vi "Acquire Data using 5772 (DRAM_200fifo_110M_globals).vi"() -> ()   [LabVIEW 2012]
uses:
  <vilib>/Platform/TimedLoop/XDataNode/XDataNode.xnode
  <vilib>/Platform/TimedLoop/XDataNode/nitl_modes.ctl
  <vilib>/Platform/TimedLoop/XDataNode/XDNodeRunTimeDep.lvlib
  <vilib>/Platform/TimedLoop/XDataNode/wakeup.ctl
  <vilib>/Platform/TimedLoop/XDataNode/timing_clust.ctl
  <vilib>/rvi/FXPMathLib/basic elements/FxpDiscreteDelay/XNode/nifxpmath_DiscreteDelay.xnode
  <userlib>/FPGA Library/Code Development/DRAM/RF-RIO/FIFO/FIFO/FPGA/FIFO.lvlib
  <userlib>/Fast OCT/Debug/Version 1/Channel Data/Data from Channel 0 and Channel 1.vi
  <userlib>/Fast OCT/Debug/Version 1/Globals/Controls.vi
panel:
  out "Record Count":u32
  out "U256s from DRAM FIFO":u32
  out "U256s to DRAM FIFO":u32
  out "Host FIFO Timed Out?":bool
  out "U64s to Host":u32
  out "U256s Acquired":u32
  in  "DRAM Arbiter Config":T1={"write grant time (clocks)"=256, "read grant time (clocks)"=256}
  in  "DRAM FIFO Depth":u8(ring)=20 items=["4"=2, "8"=3, "16"=4, "32"=5, "64"=6, "128"=7, "256"=8, "512"=9, "1024"=10, "2048"=11, "4096"=12, "8192"=13, "16384"=14, "32768"=15, "65536"=16, "131072"=17, "262144"=18, "524288"=19, "1048576"=20, "2097152"=21, "4194304"=22, "8388608"=23, "16777216"=24, "33554432"=25, "67108864"=26, "134217728"=27, "268435456"=28, "536870912"=29, "1073741824"=30, "2147483648"=31, "4294967296"=32]
  in  "Record Parameters":T2={"Load Record Parameters?"=FALSE, "Pre Trigger Samples"=2, "Post Trigger Samples"=1000, "Trigger Hold Off"=0, "Record Count"=1} {"Pre Trigger Samples" min=2}
  out "IO Module Status":T3
  out "Buffer Timed Out?":bool
  in  "Software Trigger":bool
  in  "Trigger Type":T4(ring)=enum."Software Trigger"
  in  "Arm Acquisition Engine":bool
  # "Digitial Trigger Input:\nPXI_Trig0 or DIO 0 on CB Front Panel"
  # "Interactive Mode Instructions\n1) Run the Emulation Mode VI for Stimulus\n1) Click on acq.Initiate, First to False and Then to True\n2) Click on Host Trigger"
  # "Status"
  # "Acquisition Engine"
  # "Acquisition Status"
  # "Record Parameters"
  # "Memory Configuration"
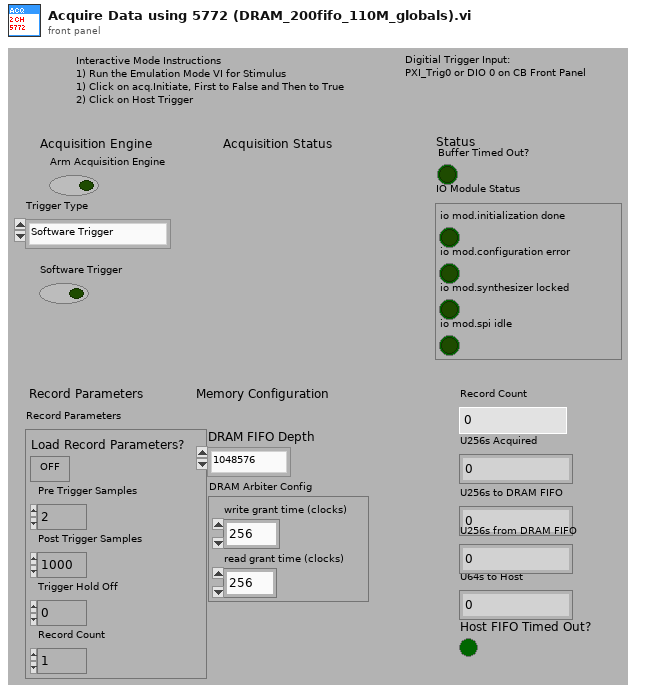
[diagram p1: front panel]
types:
  T1 = cluster{"write grant time (clocks)":u16, "read grant time (clocks)":u16}
  T2 = cluster{"Load Record Parameters?":bool, "Pre Trigger Samples":u32, "Post Trigger Samples":u32, "Trigger Hold Off":u32, "Record Count":u32}
  T3 = cluster{"io mod.initialization done":bool, "io mod.configuration error":bool, "io mod.synthesizer locked":bool, "io mod.spi idle":bool}
  T4 = enum8{"Immediate Trigger", "Software Trigger", "External Digital Trigger", "Analog Trigger"}
  T5 = typedef "XDNodeRunTimeDep.lvlib/timing_clust.ctl" = cluster{"Expected End [f-1]":u64, "Actual End [f-1]":u64, "Finished Late? [f-1]":bool, "Expected End [i-1]":u64, "Actual End [i-1]":u64, "Finished Late? [i-1]":bool, "Expected Start [i]":u64, "Actual Start [i]":u64, "Expected Start [f]":u64, "Actual Start [f]":u64, "Source Name":string, "Structure Name":string, "Period":i64, "Deadline":i64, "Offset":i64, "Start":i64, "Priority":i32, "Timeout":i32, "Mode":T6, "Wakeup Reason":T7, "Error":errorcluster, "Source Type":string, "Secondary Source Type":string, "Global End Time":u64, "Global Start Time":u64, "Frame Duration":u64, "Iteration Duration":u64, "Assigned CPU":i32, "I/O Scan Engine Mode":u32}
  T6 = typedef "XDNodeRunTimeDep.lvlib/nitl_modes.ctl" = enum32{"No Change", "Process missed periods, maintain original phase", "Discard missed periods, maintain original phase", "Process missed periods, ignore original phase", "Discard missed periods, ignore original phase"}
  T7 = typedef "XDNodeRunTimeDep.lvlib/wakeup.ctl" = enum32{"Normal", "Aborted", "Asynchronous wakeup", "Timing source error", "Timed loop error", "Timeout"}
  T8 = cluster{"fifo1 memory":refnum<k21>, "fifo2 memory":refnum<k21>}
  T9 = cluster{"Data 0":u64, "Data 1":u64, "Data 2":u64, "Data 3":u64}
  T10 = cluster{"Output":cluster{"Data 0":u64, "Data 1":u64, "Data 2":u64, "Data 3":u64}, "Output Valid":bool}
  T11 = typedef "Data Type (256).ctl" = cluster{"Bank0. High":u64, "Bank0. Low":u64, "Bank1. High":u64, "Bank1. Low":u64}
  T12 = typedef "acqEngineStates v1.ctl" = cluster{"Triggered":bool, "TrigArmed":bool, "RdyForArm":bool, "Reserved":bool}
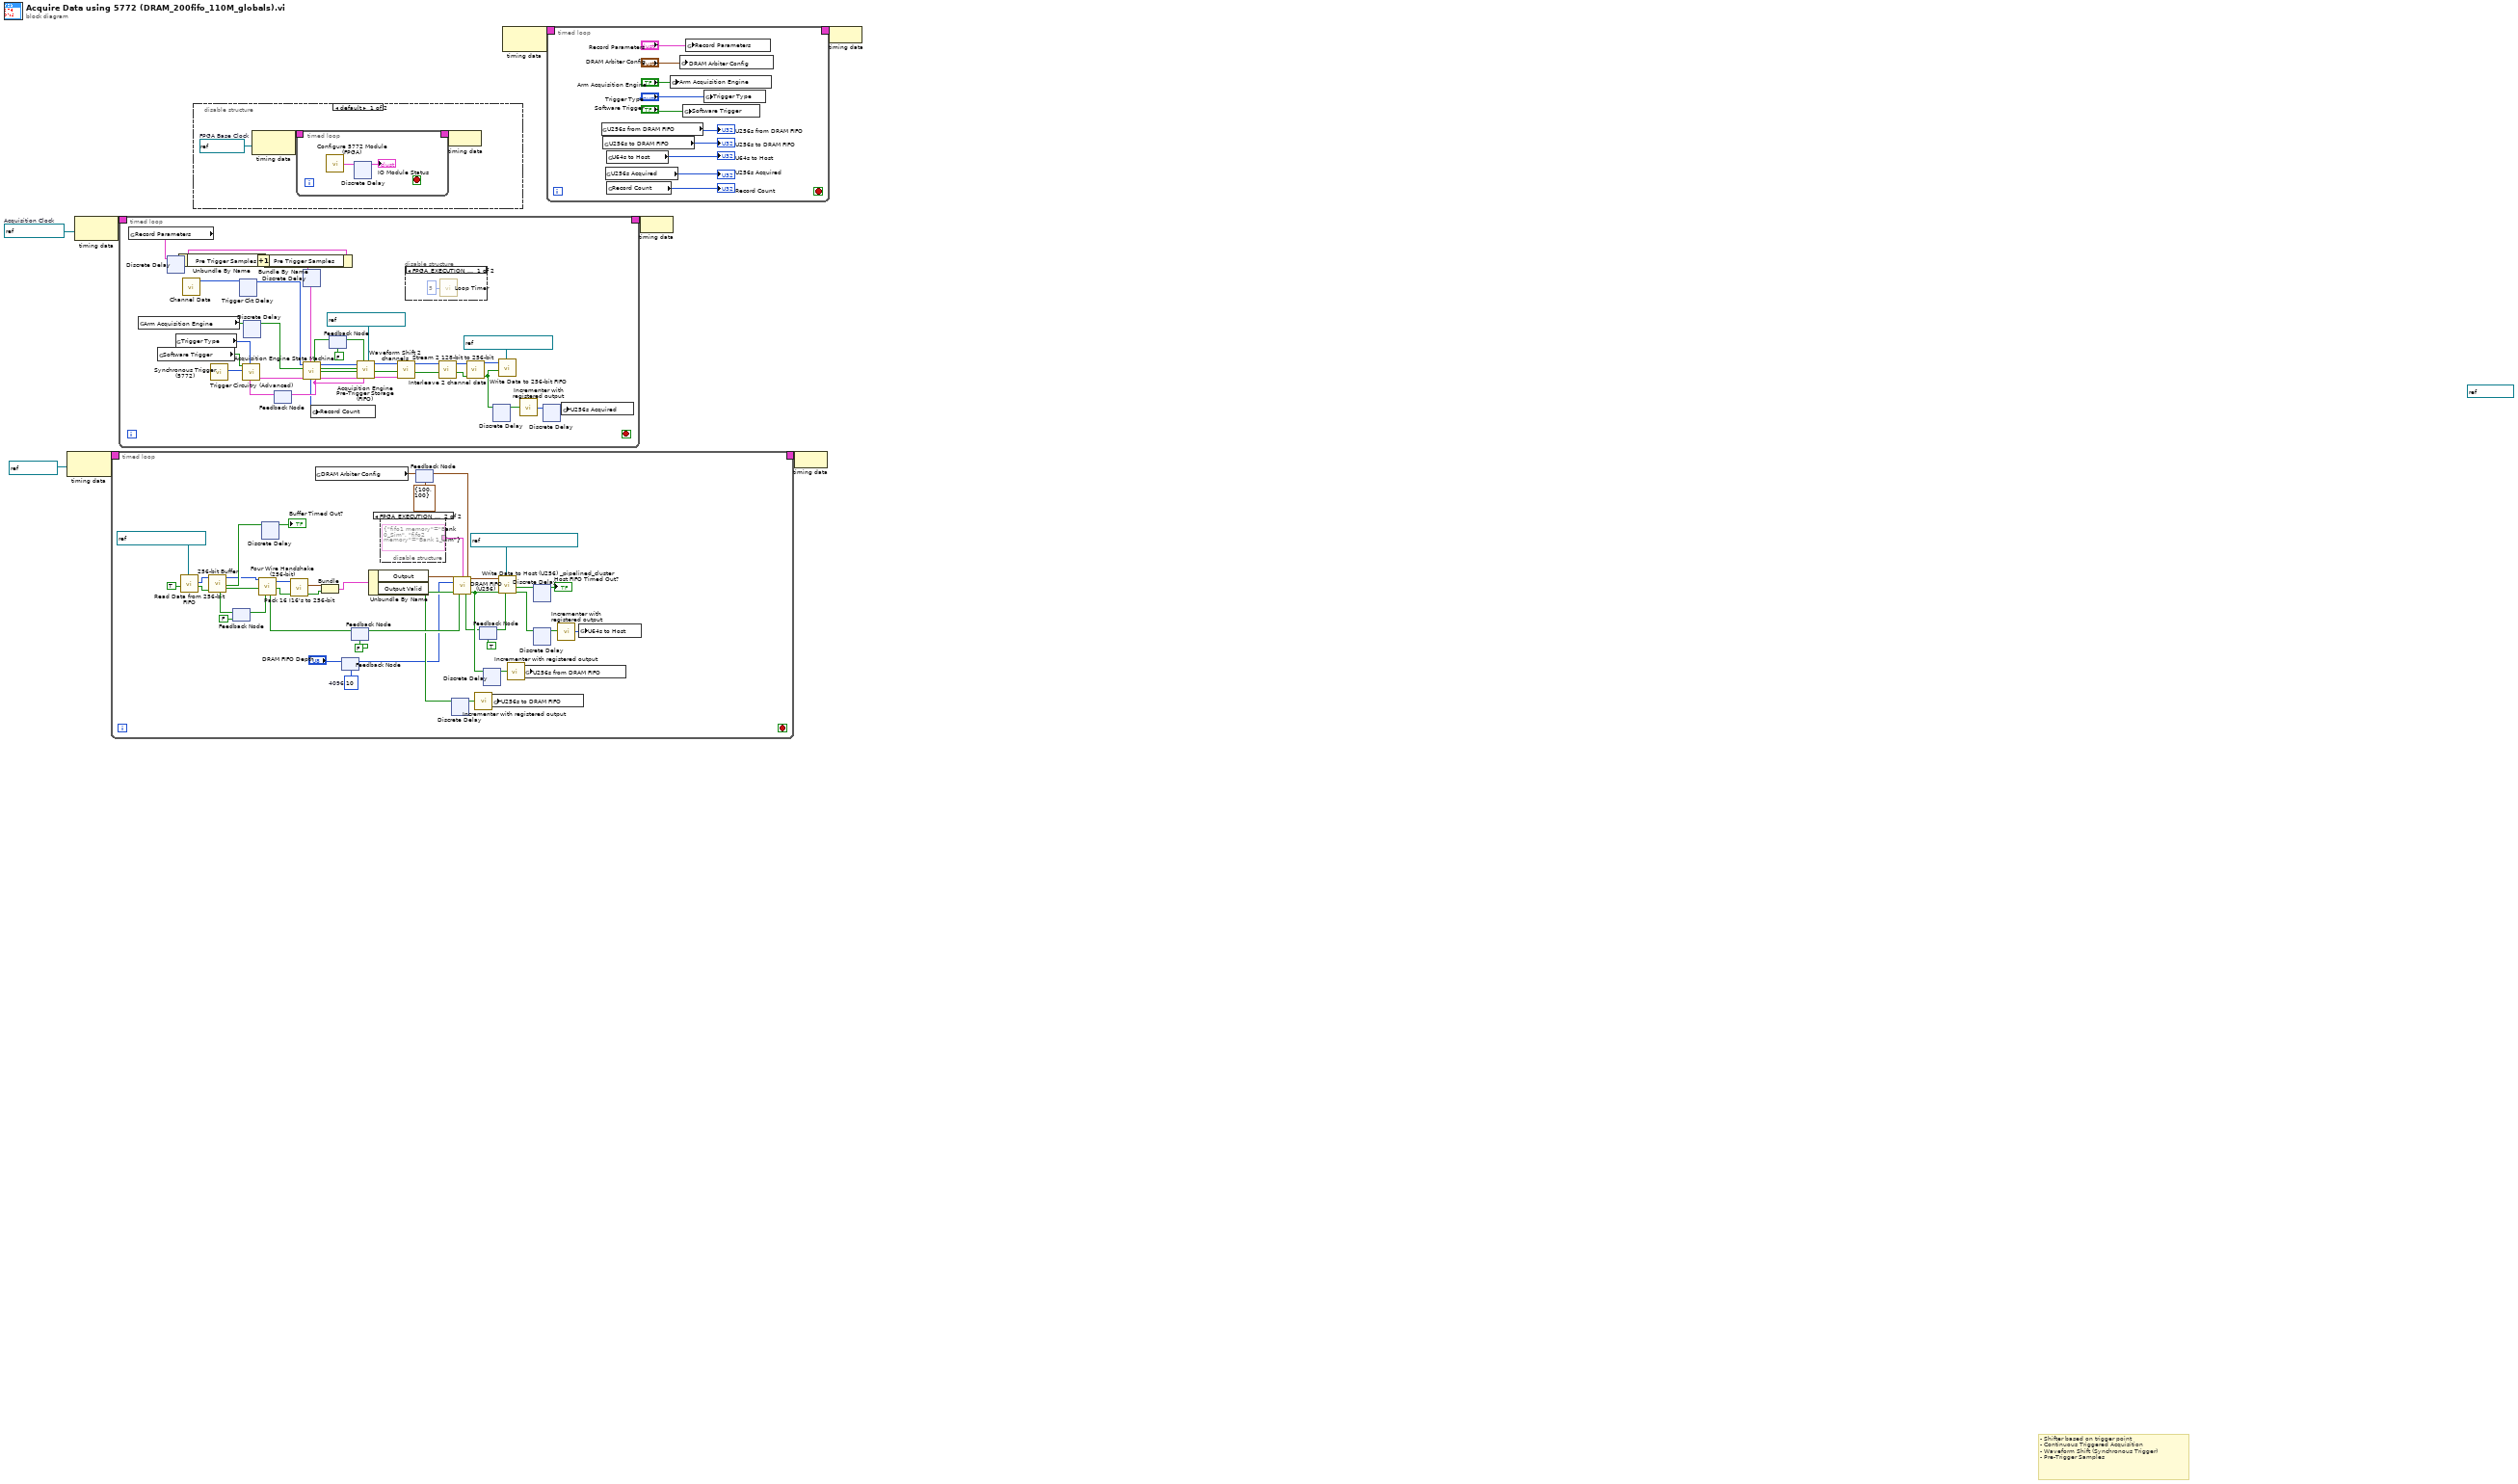
[diagram p0: block diagram]
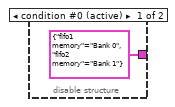
[diagram p3: hidden frame]
diagram:
  (unwired) refnum<k21> "To Host" ("FIFO In")
  w6 = refnum<k21> "ADC Clock Div 4"  # Acquisition Clock
  # "- Shifter based on trigger point\n- Continuous Triggered Acquisition\n- Waveform Shift (Synchronous Trigger)\n- Pre-Trigger Samples"
  n1 = node-c288(refnum<k21> "110MHz" ("Source Name")) -> (w5:T5)
  n2 = node-c288(w6) -> (w8:T5)
  n3 = timed-loop {
    timing: w5 -> [_]
    timing-out: [_] -> w4
    stop <- _ stop-if-true
    w26 = u8 10  # 4096
    n4 = call <userlib>:"Read Data from 256-bit FIFO.vi"("FIFO In"=refnum<k21> "FromAcqLoopU256", "Get New Data?"=TRUE) -> ("Data Valid"=w25:bool, "FIFO Data"=w24:i16[])  [unwired: 8 in]
    n5 = feedback #1(FALSE ("ready for input")) -> (w14:bool)
    n6 = call <userlib>:"256-bit Buffer.vi"("Ready for Output"=w14, "Input Valid"=w25, "Input"=w24) -> ("Output Valid"=w18:bool, "Ever Timed Out?"=w22:bool, "Output"=w17:i16[])  [unwired: 6 in]
    n7 = xnode "Discrete Delay"("D"=w22) -> ("Q"=→"Buffer Timed Out?":bool)
    n8 = global read "Controls.vi" "DRAM Arbiter Config"() -> (w12:T1)
    n9 = feedback-in #2("DRAM FIFO Depth") -> ()
    n10 = feedback #2(w26) -> (w27:u8)
    n11 = feedback #3(FALSE ("Ready for Input")) -> (w16:bool)
    n12 = call <userlib>:"Four Wire Handshake (256-bit).vi"("ready for output"=w16, "data valid"=w18, "Data In"=w17) -> ("valid out"=w19:bool, "Data Out"=w20:i16[], "ready for input"=w15:bool)  [unwired: 5 in, 1 out]
    n13 = feedback-in #1(w15) -> ()
    n14 = call <userlib>:"Pack 16 I16's to 256-bit.vi"("Data Valid"=w19, "Input"=w20) -> ("Output Valid"=w37:bool, "Output"=w38:T9)  [unwired: 7 in, 1 out]
    n15 = Bundle("Output"=w38, "Output Valid"=w37) -> (w34:T10)  [unwired: 1 in]
    n16 = Unbundle By Name(w34) -> ("Output"=w36:T9, "Output Valid"=w35:bool)
    n17 = disable-structure shown="FPGA_EXECUTION_MODE==DEV_COMPUTER_SIM_IO" {
      disable-tunnel: [T8 {"fifo1 memory"="Bank 0", "fifo2 memory"="Bank 1"} ("Memory") T8 {"fifo1 memory"="Bank 0_Sim", "fifo2 memory"="Bank 1_Sim"} ("Memory")] -> w49
      frame condition #0 (active) {
      }
      frame condition #1 {
      }
    }
    n18 = feedback-in #4(w12) -> ()
    n19 = feedback #4(T1 {"write grant time (clocks)"=100, "read grant time (clocks)"=100} ("DRAM Arbiter Config")) -> (w28:T1)
    n20 = xnode "Discrete Delay"("D"=w35) -> ("Q"=w31:bool)
    n21 = call <userlib>:"Incrementer with registered output.vi"("INC?"=w31) -> ("count"=w9:u32)  [unwired: 4 in]
    n22 = feedback #5(TRUE ("Ready For Input")) -> (w40:bool)
    n23 = call <userlib>:"DRAM FIFO (U256).vi"("Input Data"=w36, "Memory"=w49, "arbiter configuration"=w28, "fifo depth"=w27, "input valid"=w35, "ready for output"=w40) -> ("Output Data"=w45:T11, "Ready for Input"=w48:bool, "Output Valid"=w42:bool)  [unwired: 4 in, 3 out]
    n24 = feedback-in #3(w48) -> ()
    n25 = xnode "Discrete Delay"("D"=w42) -> ("Q"=w32:bool)
    n26 = global write "Controls.vi" "U256s to DRAM FIFO"(w9) -> ()
    n27 = call <userlib>:"Write Data to Host (U256) _pipelined_cluster.vi"("FIFO In"=refnum<k21> "FPGA to Host FIFO (U64)" ("FIFO Out"), "Input Valid"=w42, "Input"=w45) -> ("Valid Data to Host"=w46:bool, "Timed Out?"=w44:bool, "Ready For Input"=w41:bool)  [unwired: 5 in, 1 out]
    n28 = feedback-in #5(w41) -> ()
    n29 = call <userlib>:"Incrementer with registered output.vi"("INC?"=w32) -> ("count"=w10:u32)  [unwired: 4 in]
    n30 = global write "Controls.vi" "U256s from DRAM FIFO"(w10) -> ()
    n31 = xnode "Discrete Delay"("D"=w44) -> ("Q"=→"Host FIFO Timed Out?":bool)
    n32 = xnode "Discrete Delay"("D"=w46) -> ("Q"=w33:bool)
    n33 = call <userlib>:"Incrementer with registered output.vi"("INC?"=w33) -> ("count"=w11:u32)  [unwired: 4 in]
    n34 = global write "Controls.vi" "U64s to Host"(w11) -> ()
  }
  n35 = timed-loop {
    timing: w8 -> [_]
    timing-out: [_] -> w7
    stop <- _ stop-if-true
    n36 = global read "Controls.vi" "Record Parameters"() -> (w61:T2)
    n37 = global read "Controls.vi" "Arm Acquisition Engine"() -> (w56:bool)
    n38 = global read "Controls.vi" "Software Trigger"() -> (w57:bool)
    n39 = xnode "Discrete Delay"("D"=w61) -> ("Q"=w65:T2)
    n40 = global read "Controls.vi" "Trigger Type"() -> (w58:T4)
    n41 = Unbundle By Name(w65) -> ("Pre Trigger Samples"=w78:u32)
    n42 = call-poly <userlib>:"Channel Data.vi"() -> ("Channels Data"=w93:i16[])  [unwired: 11 in]
    n43 = call <userlib>:"Synchronous Trigger (5772).vi"() -> ("Trigger"=w84:u8)  [unwired: 9 in, 2 out]
    n44 = xnode "Trigger Ckt Delay"("D"=w93) -> ("Q"=w75:i16[])
    n45 = xnode "Discrete Delay"("D"=w56) -> ("Q"=w62:bool)
    n46 = Increment(x=w78) -> (x+1=w77:u32)
    n47 = Bundle By Name(cluster=w65, "Pre Trigger Samples"=w77) -> (w76:T2)
    n48 = feedback #6() -> (w89:T12)  [unwired: 1 in]
    n49 = call <userlib>:"Trigger Circuitry (Advanced).vi"("State Machine State"=w89, "Trigger Type"=w58, "Digital Trigger Value"=w84, "Software Trigger from Host"=w57) -> ("Trigger Info"=w82:cluster{"Trigger":bool, "Trig Offset":u8})  [unwired: 5 in, 2 out]
    n50 = xnode "Discrete Delay"("D"=w76) -> ("Q"=w64:T2)
    n51 = feedback #7(FALSE ("flushed")) -> (w87:bool)
    n52 = call <userlib>:"Acquisition Engine State Machine.vi"("Start Next Record"=w87, "Record Parameters"=w64, "Trigger Info"=w82, "Arm Acquisition Engine"=w62, "Input"=w75) -> ("Trigger Info"=w90:cluster{"Trigger":bool, "Trig Offset":u8}, "PostTrigComplete"=w91:bool, "AcqInProgress"=w81:bool, "Output"=w92:i16[], "States"=w80:T12, "Record Count"=w60:u32)  [unwired: 1 in]
    n53 = feedback-in #6(w80) -> ()
    n54 = global write "Controls.vi" "Record Count"(w60) -> ()
    n55 = call <userlib>:"Acquisition Engine Pre-Trigger Storage (FIFO).vi"("FIFO Out"=refnum<k21> "HistoryFIFOU128", "states"=w80, "Trigger Info"=w90, "PostTrigComplete"=w91, "AcqInProgress"=w81, "Input Data"=w92) -> ("Trigger Info"=w85:cluster{"Trigger":bool, "Trig Offset":u8}, "Output Valid"=w73:bool, "Output Data"=w74:i16[], "Flushed"=w88:bool)  [unwired: 2 in]
    n56 = feedback-in #7(w88) -> ()
    n57 = call <userlib>:"Waveform Shift 2 channels.vi"("Trigger Info"=w85, "Input Valid"=w73, "Input Data"=w74) -> ("Output Valid"=w72:bool, "Shifted Output Data"=w70:i16[])  [unwired: 5 in, 2 out]
    n58 = disable-structure shown="FPGA_EXECUTION_MODE==DEV_COMPUTER_SIM_IO" {
      frame condition #0 {
        n59 = call "Loop Timer"("Count(mSec)"=u32 5) -> ()  [unwired: 1 out]
      }
      frame condition #1 (active) {
      }
    }
    n60 = call <userlib>:"Interleave 2 channel data.vi"("Input Valid"=w72, "Raw Data"=w70) -> ("Output Valid"=w68:bool, "Interleaved Data"=w69:i16[])  [unwired: 8 in]
    n61 = call <userlib>:"Stream 2 128-bit to 256-bit.vi"("Input Valid"=w68, "Input Data"=w69) -> ("Output Valid"=w66:bool, "Output Data"=w67:i16[])  [unwired: 8 in]
    n62 = xnode "Discrete Delay"("D"=w66) -> ("Q"=w63:bool)
    n63 = call <userlib>:"Write Data to 256-bit FIFO.vi"("FIFO In"=refnum<k21> "FromAcqLoopU256", "Input Valid"=w66, "Data"=w67) -> ()  [unwired: 7 in, 2 out]
    n64 = call <userlib>:"Incrementer with registered output.vi"("INC?"=w63) -> ("count"=w79:u32)  [unwired: 4 in]
    n65 = xnode "Discrete Delay"("D"=w79) -> ("Q"=w59:u32)
    n66 = global write "Controls.vi" "U256s Acquired"(w59) -> ()
  }
  n67 = disable-structure shown="default" {
    frame condition #0 (active) {
      w97 = refnum<k21> "40 MHz"  # FPGA Base Clock
      n68 = node-c288(w97) -> (w99:T5)
      n69 = timed-loop {
        timing: w99 -> [_]
        timing-out: [_] -> w98
        stop <- _ stop-if-true
        n70 = call <userlib>:"Configure 5772 Module (FPGA).vi"() -> ("IO Module Status"=w101:T3)  [unwired: 5 in]
        n71 = xnode "Discrete Delay"("D"=w101) -> ("Q"=→"IO Module Status":T3)
      }
      n72 = node-c288(w98) -> ()
    }
    frame condition #1 {
    }
  }
  n73 = node-c288() -> (w2:T5)  [unwired: 1 in]
  n74 = timed-loop {
    timing: w2 -> [_]
    timing-out: [_] -> w1
    stop <- _ stop-if-true
    n75 = global read "Controls.vi" "U256s from DRAM FIFO"() -> (→"U256s from DRAM FIFO":u32)
    n76 = global read "Controls.vi" "U256s to DRAM FIFO"() -> (→"U256s to DRAM FIFO":u32)
    n77 = global read "Controls.vi" "U256s Acquired"() -> (→"U256s Acquired":u32)
    n78 = global read "Controls.vi" "U64s to Host"() -> (→"U64s to Host":u32)
    n79 = global read "Controls.vi" "Record Count"() -> (→"Record Count":u32)
    n80 = global write "Controls.vi" "Arm Acquisition Engine"("Arm Acquisition Engine") -> ()
    n81 = global write "Controls.vi" "DRAM Arbiter Config"("DRAM Arbiter Config") -> ()
    n82 = global write "Controls.vi" "Software Trigger"("Software Trigger") -> ()
    n83 = global write "Controls.vi" "Record Parameters"("Record Parameters") -> ()
    n84 = global write "Controls.vi" "Trigger Type"("Trigger Type") -> ()
  }
  n85 = node-c288(w7) -> ()
  n86 = node-c288(w4) -> ()
  n87 = node-c288(w1) -> ()
